vi "FPGA_fast cycles-2.vi"() -> ()   [LabVIEW 2010]
uses:
  fast cycles/FPGA_run-states.ctl
  <vilib>/rvi/DataTransferAndStorage/Container/XNode/niFpgaContainer.xnode
  <vilib>/eio/EIONode/EIONode.xnode
  <vilib>/rvi/eio/nirviEIOImplementation/nirviEIOImplementation.xnode
  <vilib>/rvi/eio/common/nirviEmuClasses.ctl
  <vilib>/rvi/FIFO/Fifo_Resource/nirvififoEmulationSetSize.vi
  <vilib>/rvi/DataTransferAndStorage/Container/Common/niFpgaContainerGetUniqueNameForEmu.vi
  <vilib>/rvi/Memory/Memory_Emulation/nirvimemoryEmulationManagerCache_GetValue.vi
  <vilib>/rvi/Memory/Memory_Emulation/nirvimemoryEmulationManagerCache_InsertValue.vi
  <vilib>/Utility/error.llb/Clear Errors.vi
  <vilib>/rvi/Memory/Memory_Emulation/nirvimemoryEmulationManagerCache_SetValue.vi
  <vilib>/rvi/eio/common/nirviEmuTemplateMethod_noerrors.vi
panel:
  in  "Stop seq":bool=TRUE
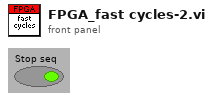
[diagram p1: front panel]
types:
  T1 = typedef "FPGA_run-states.ctl" = enum16{"stopped", "check", "reserve", "run", "release"}
  T2 = typedef "nirviEmuClasses.ctl" = enum16{"IO Read", "IO Write", "Method", "Property Read", "Property Write"}
  T3 = cluster{"Boolean array[0]":bool, "Boolean array[1]":bool, "Boolean array[2]":bool, "Boolean array[3]":bool, "Boolean array[4]":bool, "Boolean array[5]":bool, "Boolean array[6]":bool, "Boolean array[7]":bool, "Boolean array[8]":bool, "Boolean array[9]":bool, "Boolean array[10]":bool, "Boolean array[11]":bool, "Boolean array[12]":bool, "Boolean array[13]":bool, "Boolean array[14]":bool, "Boolean array[15]":bool}
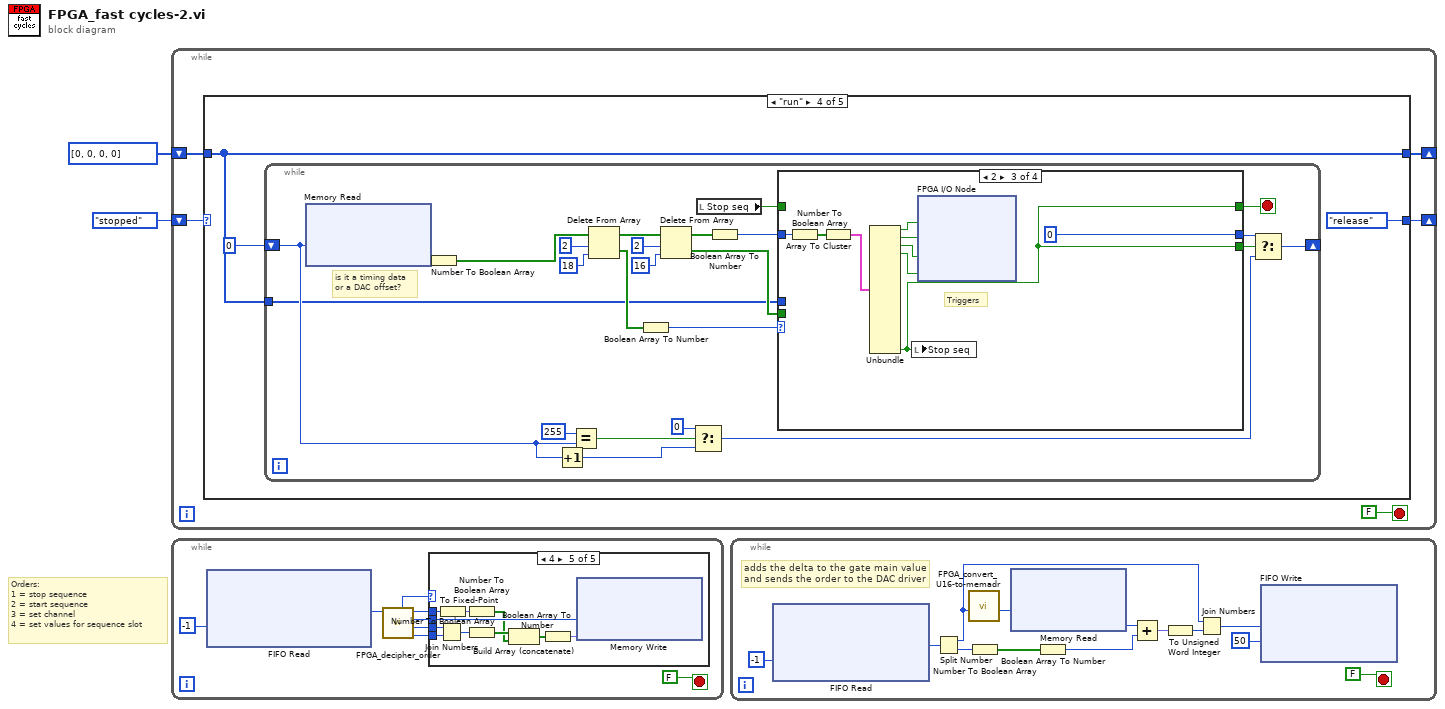
[diagram p0: block diagram]
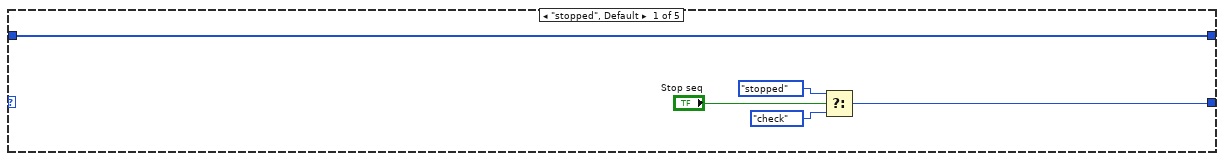
[diagram p2: hidden frame]
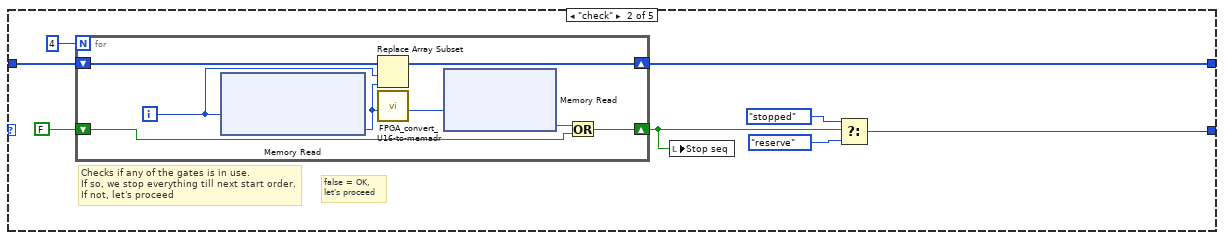
[diagram p3: hidden frame]
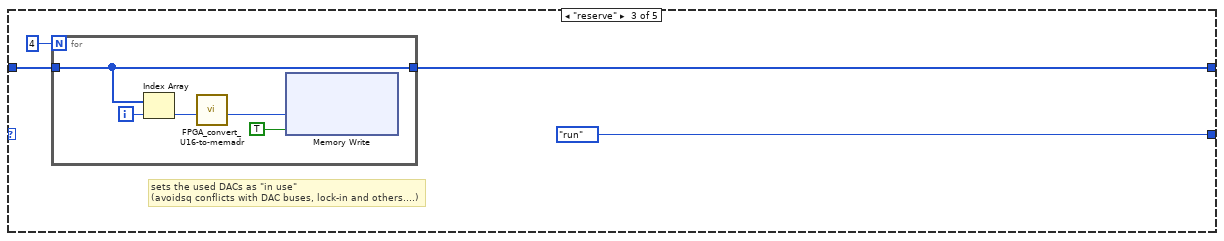
[diagram p4: hidden frame]
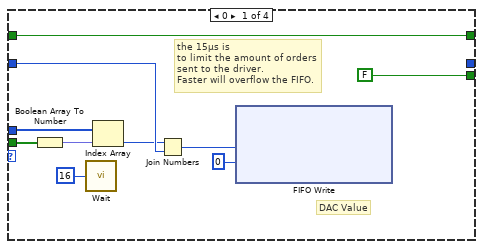
[diagram p5: hidden frame]
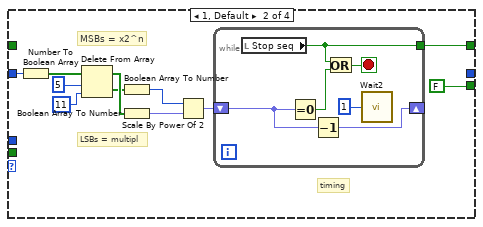
[diagram p6: hidden frame]
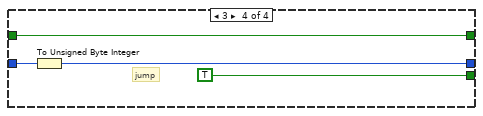
[diagram p7: hidden frame]
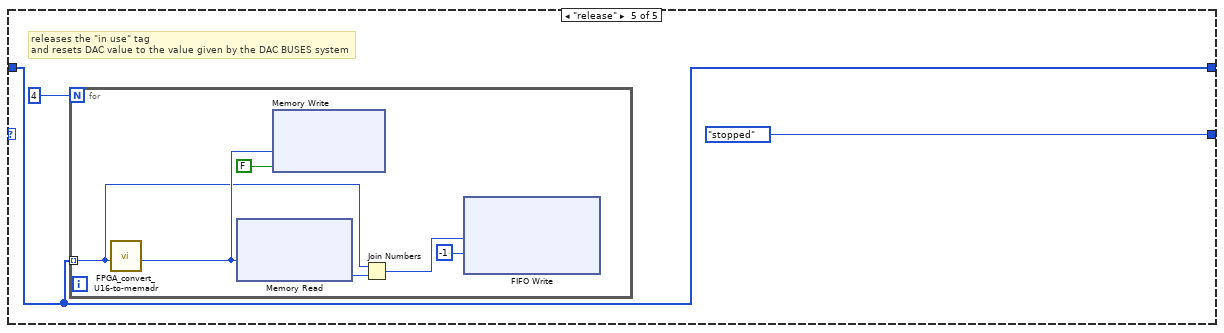
[diagram p8: hidden frame]
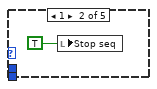
[diagram p10: hidden frame]
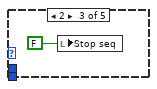
[diagram p11: hidden frame]
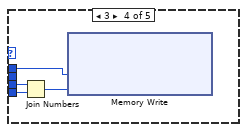
[diagram p12: hidden frame]
diagram:
  # "Orders:\n1 = stop sequence\n2 = start sequence\n3 = set channel\n4 = set values for sequence slot"
  n1 = while {
    shift-right: [w5] -> _
    shift-left: FPGA_run-states."stopped" ("run states") -> [w6]
    shift-right: [w4] -> _
    shift-left: u16[] [0, 0, 0, 0] -> [w3]
    stop <- FALSE stop-if-true
    n2 = case shown="\"run\"" w6 {
      tunnel: [w9 w16 FPGA_run-states."run" ("run states") FPGA_run-states."release" ("run states") FPGA_run-states."stopped" ("run states")] -> w5
      tunnel: [w8 w15 w282 w417 w704] -> w4
      tunnel: w3 -> [w8 w14 w284 w417 w704]
      frame "stopped", Default {
        n3 = Select(t=FPGA_run-states."stopped" ("run states"), s="Stop seq", f=FPGA_run-states."check" ("run states")) -> (s? t:f=w9:T1)
      }
      frame "check" {
        # "Checks if any of the gates is in use.\nIf so, we stop everything till next start order.\nIf not, let's proceed"
        # "false = OK,\nlet's proceed"
        n4 = for {
          N: 4 -> [_]
          shift-right: [w23] -> w13
          shift-left: FALSE ("Data") -> [w22]
          shift-right: [w21] -> w15
          shift-left: w14 -> [w28]
          i -> [w27]
          n5 = xnode ("Memory Read")("Address"=w27) -> ("Data"=w26:u16)  [unwired: 1 in, 1 out]
          n6 = Replace Array Subset(array=w28, new element=w26, index=w27) -> (w21:u16[])
          n7 = call "FPGA_convert_U16-to-memadr.vi"("Numeric"=w26) -> ("mem adr"=w25:u8)  [unwired: 10 out]
          n8 = xnode ("Memory Read")("Address"=w25) -> ("Data"=w24:bool)  [unwired: 1 in, 1 out]
          n9 = Or(x=w24, y=w22) -> (x .or. y?=w23:bool)
        }
        n10 = local write "Stop seq"(w13) -> ()
        n11 = Select(t=FPGA_run-states."stopped" ("run states"), s=w13, f=FPGA_run-states."reserve" ("run states")) -> (s? t:f=w16:T1)
      }
      frame "reserve" {
        # "sets the used DACs as \"in use\"\n(avoidsq conflicts with DAC buses, lock-in and others....)"
        n12 = for {
          N: 4 -> [_]
          tunnel: w284 -> [w285]
          tunnel: [w285] -> w282
          i -> [w287]
          n13 = Index Array(array=w285, index=w287) -> (element=w286:u16)
          n14 = call "FPGA_convert_U16-to-memadr.vi"("Numeric"=w286) -> ("mem adr"=w289:u8)  [unwired: 10 out]
          n15 = xnode ("Memory Write")("Address"=w289, "Data"=TRUE) -> ()  [unwired: 1 in, 1 out]
        }
      }
      frame "run" {
        n16 = while {
          shift-right: [w423] -> _
          shift-left: u8 0 ("t") -> [w436]
          tunnel: w417 -> [w424]
          stop <- w420 stop-if-true
          # "is it a timing data\nor a DAC offset?"
          n17 = xnode ("Memory Read")("Address"=w436) -> ("Data"=w435:fxp<+,24,24>)  [unwired: 1 in, 1 out]
          n18 = Number To Boolean Array(number=w435) -> (Boolean array=w434:bool[])
          n19 = Increment(x=w436) -> (x+1=w438:u8)
          n20 = Equal?(x=u8 255, y=w436) -> (x = y?=w440:bool)
          n21 = Delete From Array(array=w434, length=2, index=18) -> (deleted portion=w427:bool[], array with subset deleted=w431:bool[])
          n22 = Boolean Array To Number(Boolean array=w427) -> (number=w425:u8)
          n23 = Delete From Array(array=w431, length=2, index=16) -> (deleted portion=w428:bool[], array with subset deleted=w429:bool[])
          n24 = Select(t=u8 0, s=w440, f=w438) -> (s? t:f=w437:u8)
          n25 = local read "Stop seq"() -> (w419:bool)
          n26 = Boolean Array To Number(Boolean array=w429) -> (number=w418:u16)
          n27 = case shown="2" w425 {
            tunnel: w418 -> [w573 w639 w654 w699]
            tunnel: w428 -> [w577 _ _ _]
            tunnel: w424 -> [w576 _ _ _]
            tunnel: [FALSE ("Stop seq") FALSE ("Stop seq") w646 TRUE ("Stop seq")] -> w422
            tunnel: [_ _ u8 0 w701] -> w421
            tunnel: [w568 w629 w646 w700] -> w420
            tunnel: w419 -> [w568 _ _ w700]
            frame 0 {
              # "the 15µs is\nto limit the amount of orders\nsent to the driver.\nFaster will overflow the FIFO."
              # "DAC Value"
              n28 = Boolean Array To Number(Boolean array=w577) -> (number=w575:fxp<+,2,2>)
              n29 = call "Wait"("Count(uSec)"=u8 16) -> ()  [unwired: 1 out]
              n30 = Index Array(array=w576, index=w575) -> (element=w571:u16)
              n31 = Join Numbers(hi=w571, lo=w573) -> ((hi.lo)=w572:u32)
              n32 = xnode ("FIFO Write")("Element"=w572, "Timeout"=0) -> ()  [unwired: 1 in, 2 out]
            }
            frame 1, Default {
              # "MSBs = x2^n"
              # "LSBs = multipl"
              # "timing"
              n33 = Number To Boolean Array(number=w639) -> (Boolean array=w638:bool[])
              n34 = Delete From Array(array=w638, length=5 ("longueur"), index=11 ("indice")) -> (deleted portion=w634:bool[], array with subset deleted=w635:bool[])
              n35 = Boolean Array To Number ("Tableau de booléens en nombre")(Boolean array=w634) -> (number=w633:u8)
              n36 = Boolean Array To Number ("Tableau de booléens en nombre")(Boolean array=w635) -> (number=w632:fxp<+,37,37>)
              n37 = Scale By Power Of 2(n=w633, x=w632) -> (x*2^n=w631:fxp<+,37,37>)
              n38 = while {
                shift-right: [w645] -> _
                shift-left: w631 -> [w644]
                tunnel: [w641] -> w629
                stop <- w643 stop-if-true
                n39 = local read "Stop seq"() -> (w641:bool)
                n40 = Equal To 0?(x=w644) -> (x = 0?=w640:bool)
                n41 = Decrement ("Décrémenter")(x=w644) -> (x-1=w645:fxp<+,37,37>)
                n42 = Or(x=w641, y=w640) -> (x .or. y?=w643:bool)
                n43 = call "Wait2"("Count(uSec)"=u8 1) -> ()  [unwired: 1 out]
              }
            }
            frame 2 {
              # "Triggers"
              n44 = Number To Boolean Array(number=w654) -> (Boolean array=w653:bool[])
              n45 = Array To Cluster(array=w653) -> (cluster=w652:T3)
              n46 = Unbundle(w652) -> ("Boolean array[0]"=w651:bool, "Boolean array[1]"=w650:bool, "Boolean array[2]"=w649:bool, "Boolean array[3]"=w648:bool, "Boolean array[15]"=w646:bool)  [unwired: 11 out]
              n47 = local write "Stop seq"(w646) -> ()
              n48 = xnode "FPGA I/O Node"("Port9/DIO1"=w651, "Port9/DIO2"=w650, "Port9/DIO3"=w649, "Port9/DIO4"=w648) -> ()  [unwired: 4 in, 4 out]
            }
            frame 3 {
              # "jump"
              n49 = To Unsigned Byte Integer(number=w699) -> (unsigned 8bit integer=w701:u8)
            }
          }
          n50 = Select(t=w421, s=w422, f=w437) -> (s? t:f=w423:u8)
        }
      }
      frame "release" {
        # "releases the \"in use\" tag\nand resets DAC value to the value given by the DAC BUSES system"
        n51 = for {
          N: 4 -> [_]
          tunnel: w704 -> [w706] mode=indexing
          n52 = call "FPGA_convert_U16-to-memadr.vi"("Numeric"=w706) -> ("mem adr"=w710:u8)  [unwired: 10 out]
          n53 = xnode ("Memory Read")("Address"=w710) -> ("Data"=w708:u16)  [unwired: 1 in, 1 out]
          n54 = xnode ("Memory Write")("Address"=w710, "Data"=FALSE) -> ()  [unwired: 1 in, 1 out]
          n55 = Join Numbers(hi=w706, lo=w708) -> ((hi.lo)=w709:u32)
          n56 = xnode ("FIFO Write")("Element"=w709, "Timeout"=-1) -> ()  [unwired: 1 in, 2 out]
        }
      }
    }
  }
  n57 = while {
    stop <- FALSE stop-if-true
    n58 = xnode ("FIFO Read")("Timeout"=-1) -> ("Element"=w1019:u64)  [unwired: 1 in, 2 out]
    n59 = call "FPGA_decipher_order.vi"("order in"=w1019) -> ("data 1"=w1018:u8, "data 2"=w1017:u8, "data 3"=w1015:u8, "data 4"=w1016:u8, "order out"=w1014:u8)  [unwired: 6 out]
    n60 = case shown="4" w1014 {
      tunnel: w1018 -> [_ _ _ w1076 w1212]
      tunnel: w1017 -> [_ _ _ w1077 w1211]
      tunnel: w1016 -> [_ _ _ w1078 w1209]
      tunnel: w1015 -> [_ _ _ _ w1213]
      frame 0, Default {
      }
      frame 1 {
        n61 = local write "Stop seq"(TRUE ("Stop seq")) -> ()
      }
      frame 2 {
        n62 = local write "Stop seq"(FALSE ("Stop seq")) -> ()
      }
      frame 3 {
        n63 = Join Numbers(hi=w1077, lo=w1076) -> ((hi.lo)=w1075:u16)
        n64 = xnode ("Memory Write")("Address"=w1078, "Data"=w1075) -> ()  [unwired: 1 in, 1 out]
      }
      frame 4 {
        n65 = Join Numbers(hi=w1211, lo=w1212) -> ((hi.lo)=w1210:u16)
        n66 = To Fixed-Point(number=w1209) -> (fixed-point=w1208:fxp<+,4,4>)  [unwired: 1 out]
        n67 = Number To Boolean Array(number=w1208) -> (Boolean array=w1206:bool[])
        n68 = Number To Boolean Array(number=w1210) -> (Boolean array=w1207:bool[])
        n69 = Build Array (concatenate)(w1207, w1206) -> (w1205:bool[])
        n70 = Boolean Array To Number(Boolean array=w1205) -> (number=w1204:fxp<+,20,20>)
        n71 = xnode ("Memory Write")("Address"=w1213, "Data"=w1204) -> ()  [unwired: 1 in, 1 out]
      }
    }
  }
  n72 = while {
    stop <- FALSE stop-if-true
    # "adds the delta to the gate main value\nand sends the order to the DAC driver"
    n73 = xnode ("FIFO Read")("Timeout"=-1) -> ("Element"=w1350:u32)  [unwired: 1 in, 2 out]
    n74 = Split Number(x=w1350) -> (hi(x)=w1340:u16, lo(x)=w1342:u16)
    n75 = call "FPGA_convert_U16-to-memadr.vi"("Numeric"=w1340) -> ("mem adr"=w1341:u8)  [unwired: 10 out]
    n76 = Number To Boolean Array(number=w1342) -> (Boolean array=w1347:bool[])
    n77 = xnode ("Memory Read")("Address"=w1341) -> ("Data"=w1349:u16)  [unwired: 1 in, 1 out]
    n78 = Boolean Array To Number(Boolean array=w1347) -> (number=w1346:i16)
    n79 = Add(x=w1349, y=w1346) -> (x+y=w1345:fxp<+,16,16>)
    n80 = To Unsigned Word Integer(number=w1345) -> (unsigned 16bit integer=w1343:u16)
    n81 = Join Numbers(hi=w1340, lo=w1343) -> ((hi.lo)=w1344:u32)
    n82 = xnode ("FIFO Write")("Element"=w1344, "Timeout"=50) -> ()  [unwired: 1 in, 2 out]
  }
